vi "map_trap_switch_Stiffback.vi"() -> ()   [LabVIEW 2011]
panel:
  in  "KILL":bool
  in  "PAUSE":bool
  in  "RESUME":bool
  in  "QUIT":bool
  in  "up done":bool
  in  "z up":bool
  in  "Done":bool
  in  "z piastra":bool
  in  "y piastra":bool
  in  "x piastra":bool
  in  "goto y pos":bool
  in  "goto x pos":bool
  in  "Panello o piastre?":bool
  in  "End":bool
  in  "zero z - end":bool
  in  "zero x - end":bool
  in  "zero y - end":bool
  in  "goto z pos":bool
  in  "positioning done":bool
  out "output":string
  out "command":string
  in  "zero done":bool
  in  "zero z":bool
  in  "zero x":bool
  in  "zero y":bool
  # "Comandi di emergenza"
  # "Mappatura a trapezio \nper il pannello e le piastre\nSU STIFFBACK"
  # "In alto: TRUE ---> Panello"
  # "In basso: FALSE ---> Piastre"
  # "Posiziono in zero"
  # "Vado sulla piastra \ne azzero"
  # "Alzo il comparatore"
  # "Vado in posizione"
  # "Ritorno a zero"
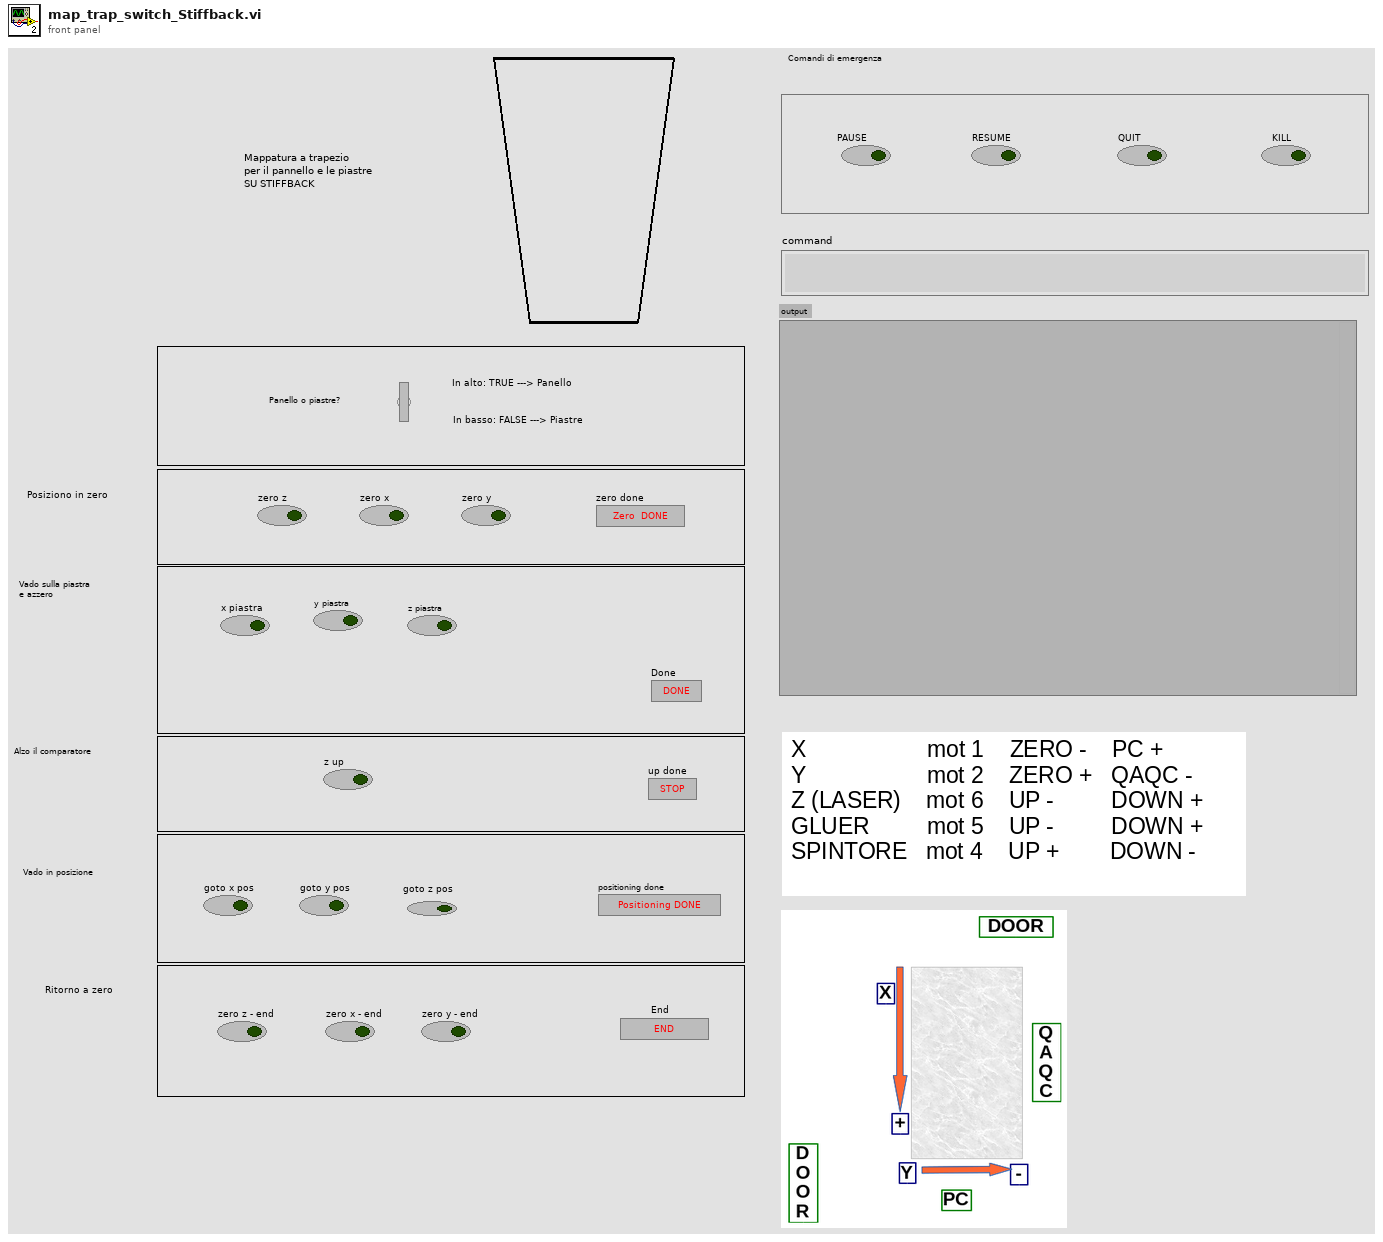
[diagram p1: front panel]
types:
  T1 = enum8{"Enabled", "Disabled", "Disabled and Grayed Out"}
  T2 = enum16{"open", "replace", "create", "open or create", "replace or create", "replace or create with confirmation"}
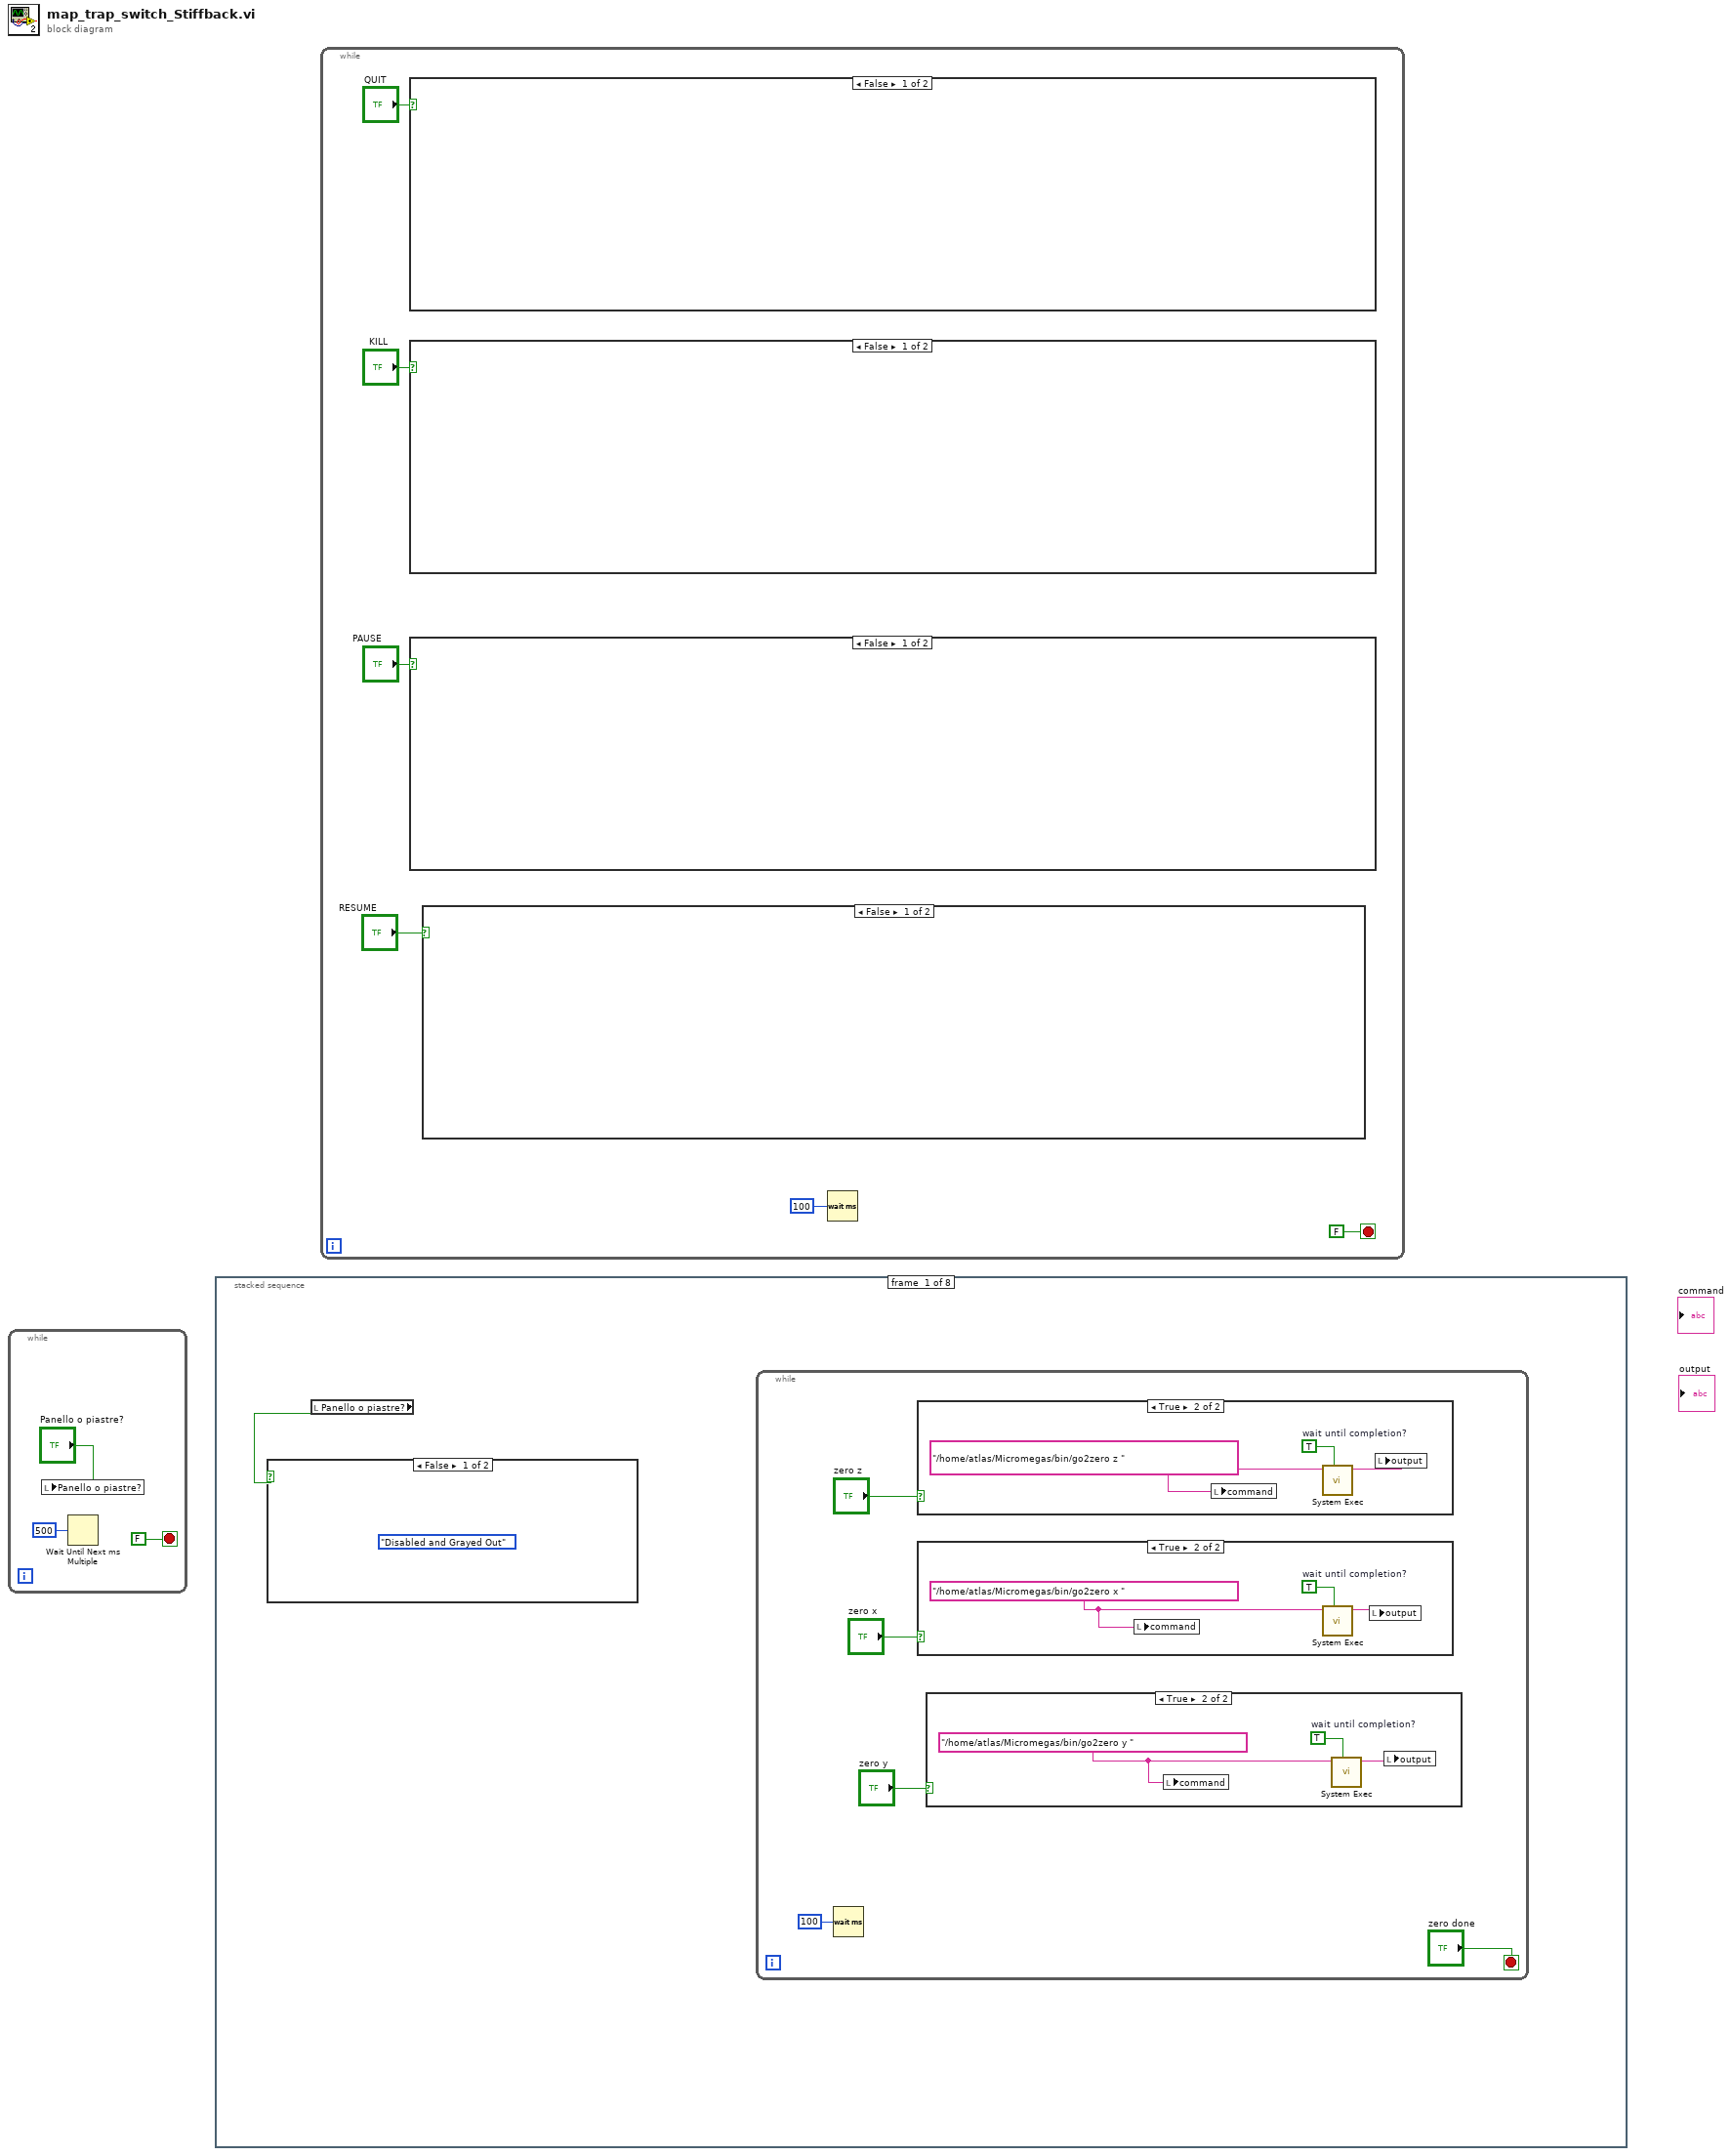
[diagram p0: block diagram]
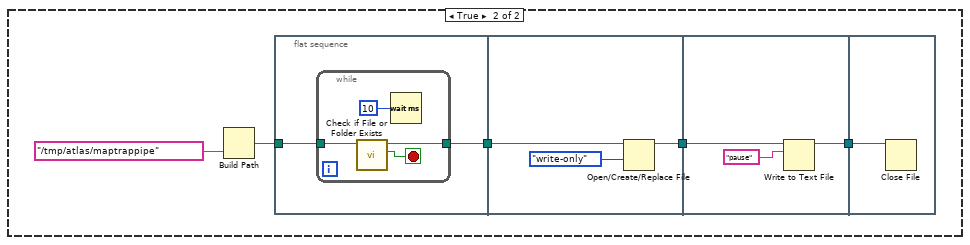
[diagram p2: hidden frame]
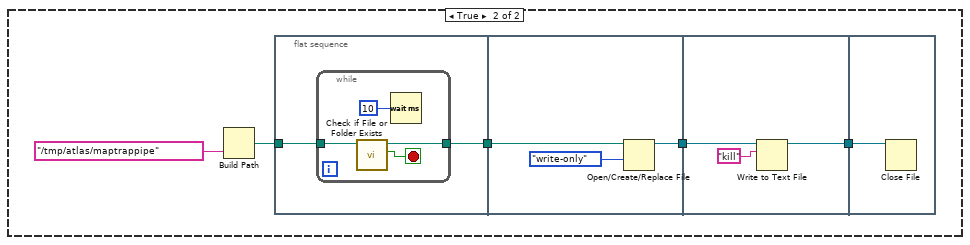
[diagram p3: hidden frame]
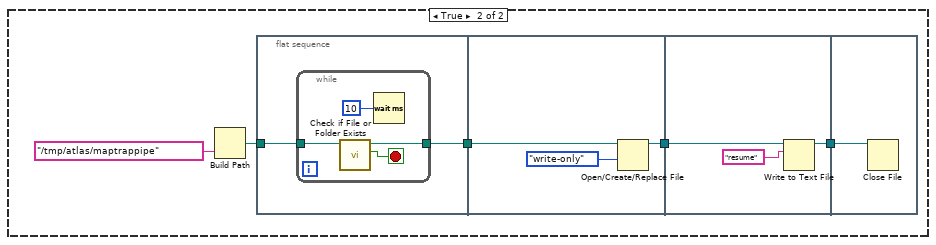
[diagram p4: hidden frame]
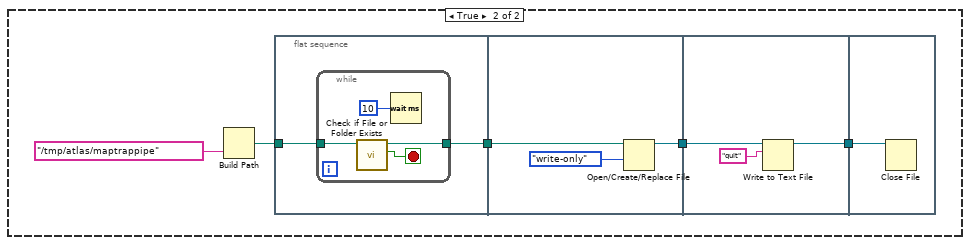
[diagram p5: hidden frame]
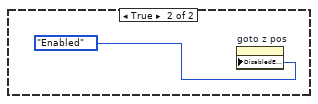
[diagram p6: hidden frame]
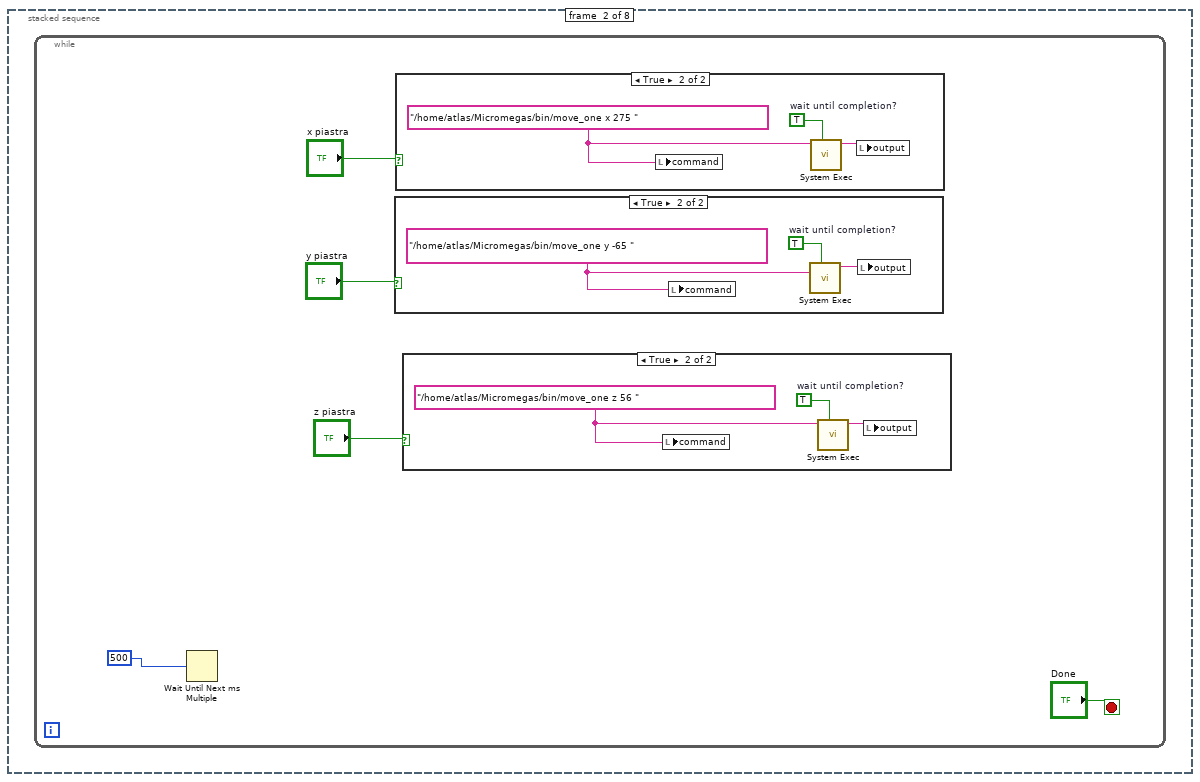
[diagram p10: hidden frame]
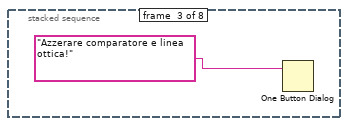
[diagram p14: hidden frame]
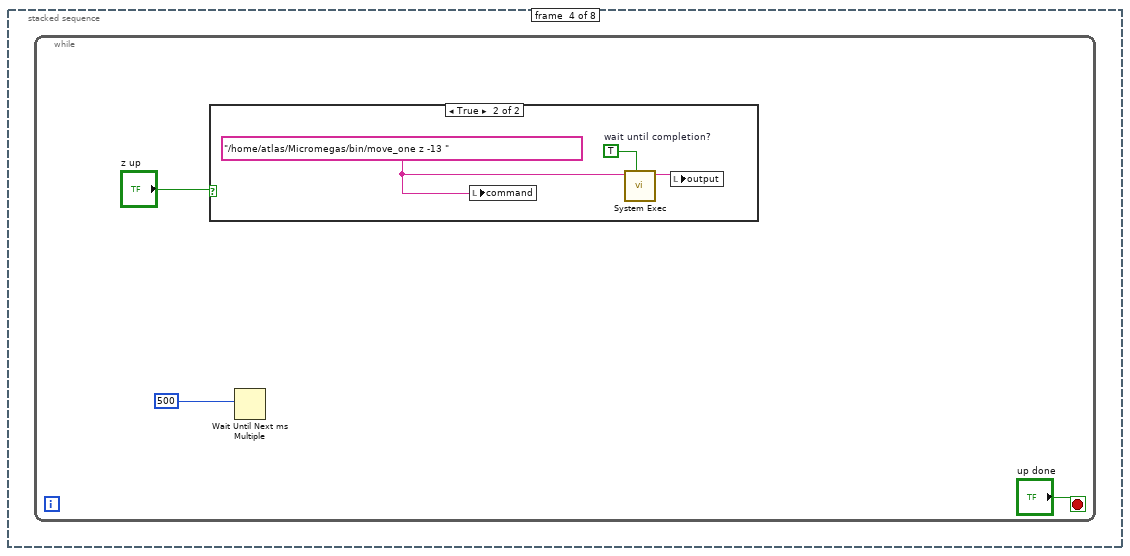
[diagram p15: hidden frame]
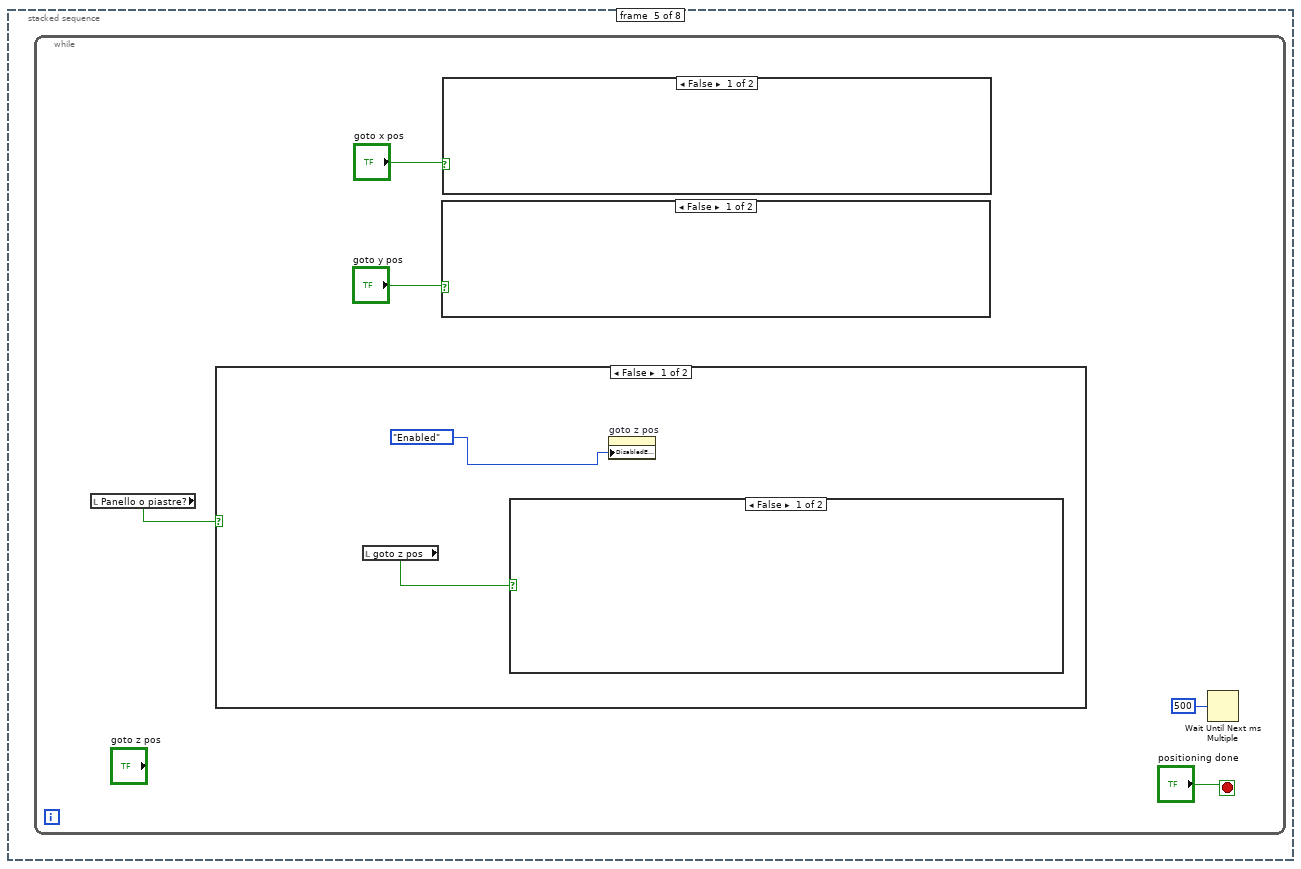
[diagram p17: hidden frame]
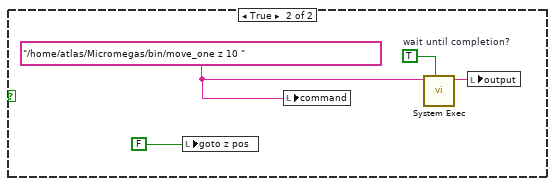
[diagram p18: hidden frame]
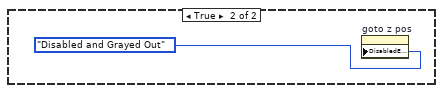
[diagram p19: hidden frame]
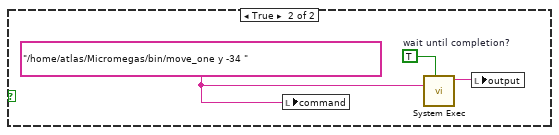
[diagram p20: hidden frame]
diagram:
  n1 = while {
    stop <- FALSE stop-if-true
    n2 = local write "Panello o piastre?"("Panello o piastre?") -> ()
    n3 = Wait Until Next ms Multiple(millisecond multiple=u32 500) -> ()  [unwired: 1 out]
  }
  n4 = stacked-sequence {
    frame #0 {
      n5 = local read "Panello o piastre?"() -> (w4:bool)
      n6 = case shown="False" w4 {
        frame False {
          (unwired) T1."Disabled and Grayed Out" ("Disabled")
        }
        frame True {
          n7 = property on="goto z pos" class="Bool (strict)"("DisabledEnum"=T1."Enabled" ("Disabled")) -> ()  [unwired: 2 in, 2 out]
        }
      }
      n8 = while {
        stop <- "zero done" stop-if-true
        n9 = Wait (ms)(milliseconds to wait=u32 100) -> ()  [unwired: 1 out]
        n10 = case shown="True" "zero z" {
          frame False {
          }
          frame True {
            w18 = "/home/atlas/Micromegas/bin/go2zero z " ("string")
            w19 = TRUE  # wait until completion?
            n11 = local write "command"(w18) -> ()
            n12 = call <vilib>:"System Exec.vi"("wait until completion? (T)"=w19, "command line"=w18) -> ("standard output"=w17:string)  [unwired: 6 in, 3 out]
            n13 = local write "output"(w17) -> ()
          }
        }
        n14 = case shown="True" "zero x" {
          frame False {
          }
          frame True {
            w15 = "/home/atlas/Micromegas/bin/go2zero x " ("string")
            w16 = TRUE  # wait until completion?
            n15 = local write "command"(w15) -> ()
            n16 = call <vilib>:"System Exec.vi"("wait until completion? (T)"=w16, "command line"=w15) -> ("standard output"=w14:string)  [unwired: 6 in, 3 out]
            n17 = local write "output"(w14) -> ()
          }
        }
        n18 = case shown="True" "zero y" {
          frame False {
          }
          frame True {
            w12 = "/home/atlas/Micromegas/bin/go2zero y " ("string")
            w13 = TRUE  # wait until completion?
            n19 = local write "command"(w12) -> ()
            n20 = call <vilib>:"System Exec.vi"("wait until completion? (T)"=w13, "command line"=w12) -> ("standard output"=w11:string)  [unwired: 6 in, 3 out]
            n21 = local write "output"(w11) -> ()
          }
        }
      }
    }
    frame #1 {
      n22 = while {
        stop <- "Done" stop-if-true
        n23 = Wait Until Next ms Multiple(millisecond multiple=u32 500 ("millisecond timer value")) -> ()  [unwired: 1 out]
        n24 = case shown="True" "y piastra" {
          frame False {
          }
          frame True {
            w28 = "/home/atlas/Micromegas/bin/move_one y -65 " ("string")
            w30 = TRUE  # wait until completion?
            n25 = local write "command"(w28) -> ()
            n26 = call <vilib>:"System Exec.vi"("wait until completion? (T)"=w30, "command line"=w28) -> ("standard output"=w29:string)  [unwired: 6 in, 3 out]
            n27 = local write "output"(w29) -> ()
          }
        }
        n28 = case shown="True" "x piastra" {
          frame False {
          }
          frame True {
            w31 = "/home/atlas/Micromegas/bin/move_one x 275 " ("string")
            w33 = TRUE  # wait until completion?
            n29 = local write "command"(w31) -> ()
            n30 = call <vilib>:"System Exec.vi"("wait until completion? (T)"=w33, "command line"=w31) -> ("standard output"=w32:string)  [unwired: 6 in, 3 out]
            n31 = local write "output"(w32) -> ()
          }
        }
        n32 = case shown="True" "z piastra" {
          frame False {
          }
          frame True {
            w25 = "/home/atlas/Micromegas/bin/move_one z 56 " ("string")
            w27 = TRUE  # wait until completion?
            n33 = local write "command"(w25) -> ()
            n34 = call <vilib>:"System Exec.vi"("wait until completion? (T)"=w27, "command line"=w25) -> ("standard output"=w26:string)  [unwired: 6 in, 3 out]
            n35 = local write "output"(w26) -> ()
          }
        }
      }
    }
    frame #2 {
      n36 = One Button Dialog(message="Azzerare comparatore e linea ottica!") -> ()  [unwired: 1 in, 1 out]
    }
    frame #3 {
      n37 = while {
        stop <- "up done" stop-if-true
        n38 = case shown="True" "z up" {
          frame False {
          }
          frame True {
            w38 = "/home/atlas/Micromegas/bin/move_one z -13 " ("string")
            w40 = TRUE  # wait until completion?
            n39 = local write "command"(w38) -> ()
            n40 = call <vilib>:"System Exec.vi"("wait until completion? (T)"=w40, "command line"=w38) -> ("standard output"=w39:string)  [unwired: 6 in, 3 out]
            n41 = local write "output"(w39) -> ()
          }
        }
        n42 = Wait Until Next ms Multiple(millisecond multiple=u32 500 ("millisecond timer value")) -> ()  [unwired: 1 out]
      }
    }
    frame #4 {
      n43 = while {
        stop <- "positioning done" stop-if-true
        n44 = local read "Panello o piastre?"() -> (w41:bool)
        n45 = case shown="False" w41 {
          frame False {
            n46 = local read "goto z pos"() -> (w47:bool)
            n47 = case shown="False" w47 {
              frame False {
              }
              frame True {
                w49 = "/home/atlas/Micromegas/bin/move_one z 10 " ("string")
                w51 = TRUE  # wait until completion?
                n48 = local write "goto z pos"(FALSE ("goto z pos")) -> ()
                n49 = local write "command"(w49) -> ()
                n50 = call <vilib>:"System Exec.vi"("wait until completion? (T)"=w51, "command line"=w49) -> ("standard output"=w50:string)  [unwired: 6 in, 3 out]
                n51 = local write "output"(w50) -> ()
              }
            }
            n52 = property on="goto z pos" class="Bool (strict)"("DisabledEnum"=T1."Enabled" ("Disabled")) -> ()  [unwired: 2 in, 2 out]
          }
          frame True {
            n53 = property on="goto z pos" class="Bool (strict)"("DisabledEnum"=T1."Disabled and Grayed Out" ("Disabled")) -> ()  [unwired: 2 in, 2 out]
          }
        }
        n54 = case shown="False" "goto y pos" {
          frame False {
          }
          frame True {
            w53 = "/home/atlas/Micromegas/bin/move_one y -34 " ("string")
            w55 = TRUE  # wait until completion?
            n55 = local write "command"(w53) -> ()
            n56 = call <vilib>:"System Exec.vi"("wait until completion? (T)"=w55, "command line"=w53) -> ("standard output"=w54:string)  [unwired: 6 in, 3 out]
            n57 = local write "output"(w54) -> ()
          }
        }
        n58 = case shown="False" "goto x pos" {
          frame False {
          }
          frame True {
            w56 = "/home/atlas/Micromegas/bin/move_one x 34 " ("string")
            w58 = TRUE  # wait until completion?
            n59 = local write "command"(w56) -> ()
            n60 = call <vilib>:"System Exec.vi"("wait until completion? (T)"=w58, "command line"=w56) -> ("standard output"=w57:string)  [unwired: 6 in, 3 out]
            n61 = local write "output"(w57) -> ()
          }
        }
        n62 = Wait Until Next ms Multiple(millisecond multiple=u32 500) -> ()  [unwired: 1 out]
      }
    }
    frame #5 {
      n63 = flat-sequence {
        frame #0 {
          n64 = Open/Create/Replace File(file path (use dialog)=path "/tmp/map_trap.tmp", operation (0:open)=T2."open or create") -> ()  [unwired: 4 in, 3 out]
          n65 = call <vilib>:"System Exec.vi"("wait until completion? (T)"=FALSE, "command line"="gnome-terminal -e \"tail -f /tmp/map_trap.tmp\"") -> ()  [unwired: 6 in, 4 out]
        }
        frame #1 {
          w69 = TRUE  # wait until completion?
          n66 = Concatenate Strings("/home/atlas/Micromegas/bin/map_trap  " ("string"), "" ("string"), "-w 2160 1120 -x 80 20 -y 80 20 -t 3 10" ("string"), "  | tee /tmp/map_trap.tmp" ("string")) -> (w64:string)
          n67 = local write "command"(w64) -> ()
          n68 = call <vilib>:"System Exec.vi"("wait until completion? (T)"=w69, "command line"=w64) -> ("standard output"=w63:string)  [unwired: 6 in, 3 out]
          n69 = local write "output"(w63) -> ()
        }
      }
    }
    frame #6 {
      n70 = while {
        stop <- "End" stop-if-true
        n71 = Wait (ms)(milliseconds to wait=u32 100) -> ()  [unwired: 1 out]
        n72 = case shown="True" "zero z - end" {
          frame False {
          }
          frame True {
            w82 = "/home/atlas/Micromegas/bin/go2zero z " ("string")
            w83 = TRUE  # wait until completion?
            n73 = local write "command"(w82) -> ()
            n74 = call <vilib>:"System Exec.vi"("wait until completion? (T)"=w83, "command line"=w82) -> ("standard output"=w81:string)  [unwired: 6 in, 3 out]
            n75 = local write "output"(w81) -> ()
          }
        }
        n76 = case shown="True" "zero x - end" {
          frame False {
          }
          frame True {
            w79 = "/home/atlas/Micromegas/bin/go2zero x " ("string")
            w80 = TRUE  # wait until completion?
            n77 = local write "command"(w79) -> ()
            n78 = call <vilib>:"System Exec.vi"("wait until completion? (T)"=w80, "command line"=w79) -> ("standard output"=w78:string)  [unwired: 6 in, 3 out]
            n79 = local write "output"(w78) -> ()
          }
        }
        n80 = case shown="True" "zero y - end" {
          frame False {
          }
          frame True {
            w76 = "/home/atlas/Micromegas/bin/go2zero y " ("string")
            w77 = TRUE  # wait until completion?
            n81 = local write "command"(w76) -> ()
            n82 = call <vilib>:"System Exec.vi"("wait until completion? (T)"=w77, "command line"=w76) -> ("standard output"=w75:string)  [unwired: 6 in, 3 out]
            n83 = local write "output"(w75) -> ()
          }
        }
      }
    }
    frame #7 {
      n84 = One Button Dialog(message="Per comodita`, rinominare il file (non verra` comunque sovrascritto)") -> ()  [unwired: 1 in, 1 out]
    }
  }
  n85 = while {
    stop <- FALSE stop-if-true
    n86 = case shown="False" "QUIT" {
      frame False {
      }
      frame True {
        n87 = Build Path(name or relative path="/tmp/atlas/maptrappipe" ("string")) -> (appended path=w145:path)  [unwired: 1 in]
        n88 = flat-sequence {
          tunnel: [w151] -> w149
          tunnel: w145 -> [w150]
          tunnel: w149 -> [w158]
          tunnel: [w156] -> w148
          tunnel: w148 -> [w161]
          tunnel: [w160] -> w147
          tunnel: w147 -> [w162]
          frame #0 {
            n89 = while {
              tunnel: [w153] -> w151
              tunnel: w150 -> [w152]
              stop <- w154 stop-if-true
              n90 = call <vilib>:"Check if File or Folder Exists.vi"("path"=w152) -> ("file or folder exists?"=w154:bool, "dup path"=w153:path)  [unwired: 8 in, 1 out]
              n91 = Wait (ms)(milliseconds to wait=u32 10) -> ()  [unwired: 1 out]
            }
          }
          frame #1 {
            n92 = Open/Create/Replace File(file path (use dialog)=w158, access (0:read/write)=enum16{"read/write", "read-only", "write-only"}."write-only") -> (refnum out=w156:refnum<file>)  [unwired: 4 in, 2 out]
          }
          frame #2 {
            n93 = Write to Text File(file (use dialog)=w161, text="quit") -> (refnum out=w160:refnum<file>)  [unwired: 2 in, 2 out]
          }
          frame #3 {
            n94 = Close File(refnum=w162) -> ()  [unwired: 1 in, 2 out]
          }
        }
      }
    }
    n95 = case shown="False" "KILL" {
      frame False {
      }
      frame True {
        n96 = Build Path(name or relative path="/tmp/atlas/maptrappipe" ("string")) -> (appended path=w109:path)  [unwired: 1 in]
        n97 = flat-sequence {
          tunnel: [w115] -> w113
          tunnel: w109 -> [w114]
          tunnel: w113 -> [w122]
          tunnel: [w120] -> w112
          tunnel: w112 -> [w125]
          tunnel: [w124] -> w111
          tunnel: w111 -> [w126]
          frame #0 {
            n98 = while {
              tunnel: [w117] -> w115
              tunnel: w114 -> [w116]
              stop <- w118 stop-if-true
              n99 = call <vilib>:"Check if File or Folder Exists.vi"("path"=w116) -> ("file or folder exists?"=w118:bool, "dup path"=w117:path)  [unwired: 8 in, 1 out]
              n100 = Wait (ms)(milliseconds to wait=u32 10) -> ()  [unwired: 1 out]
            }
          }
          frame #1 {
            n101 = Open/Create/Replace File(file path (use dialog)=w122, access (0:read/write)=enum16{"read/write", "read-only", "write-only"}."write-only") -> (refnum out=w120:refnum<file>)  [unwired: 4 in, 2 out]
          }
          frame #2 {
            n102 = Write to Text File(file (use dialog)=w125, text="kill") -> (refnum out=w124:refnum<file>)  [unwired: 2 in, 2 out]
          }
          frame #3 {
            n103 = Close File(refnum=w126) -> ()  [unwired: 1 in, 2 out]
          }
        }
      }
    }
    n104 = case shown="False" "PAUSE" {
      frame False {
      }
      frame True {
        n105 = Build Path(name or relative path="/tmp/atlas/maptrappipe" ("string")) -> (appended path=w91:path)  [unwired: 1 in]
        n106 = flat-sequence {
          tunnel: [w97] -> w95
          tunnel: w91 -> [w96]
          tunnel: w95 -> [w104]
          tunnel: [w102] -> w94
          tunnel: w94 -> [w107]
          tunnel: [w106] -> w93
          tunnel: w93 -> [w108]
          frame #0 {
            n107 = while {
              tunnel: [w99] -> w97
              tunnel: w96 -> [w98]
              stop <- w100 stop-if-true
              n108 = call <vilib>:"Check if File or Folder Exists.vi"("path"=w98) -> ("file or folder exists?"=w100:bool, "dup path"=w99:path)  [unwired: 8 in, 1 out]
              n109 = Wait (ms)(milliseconds to wait=u32 10) -> ()  [unwired: 1 out]
            }
          }
          frame #1 {
            n110 = Open/Create/Replace File(file path (use dialog)=w104, access (0:read/write)=enum16{"read/write", "read-only", "write-only"}."write-only") -> (refnum out=w102:refnum<file>)  [unwired: 4 in, 2 out]
          }
          frame #2 {
            n111 = Write to Text File(file (use dialog)=w107, text="pause") -> (refnum out=w106:refnum<file>)  [unwired: 2 in, 2 out]
          }
          frame #3 {
            n112 = Close File(refnum=w108) -> ()  [unwired: 1 in, 2 out]
          }
        }
      }
    }
    n113 = case shown="False" "RESUME" {
      frame False {
      }
      frame True {
        n114 = Build Path(name or relative path="/tmp/atlas/maptrappipe" ("string")) -> (appended path=w127:path)  [unwired: 1 in]
        n115 = flat-sequence {
          tunnel: [w133] -> w131
          tunnel: w127 -> [w132]
          tunnel: w131 -> [w140]
          tunnel: [w138] -> w130
          tunnel: w130 -> [w143]
          tunnel: [w142] -> w129
          tunnel: w129 -> [w144]
          frame #0 {
            n116 = while {
              tunnel: [w135] -> w133
              tunnel: w132 -> [w134]
              stop <- w136 stop-if-true
              n117 = call <vilib>:"Check if File or Folder Exists.vi"("path"=w134) -> ("file or folder exists?"=w136:bool, "dup path"=w135:path)  [unwired: 8 in, 1 out]
              n118 = Wait (ms)(milliseconds to wait=u32 10) -> ()  [unwired: 1 out]
            }
          }
          frame #1 {
            n119 = Open/Create/Replace File(file path (use dialog)=w140, access (0:read/write)=enum16{"read/write", "read-only", "write-only"}."write-only") -> (refnum out=w138:refnum<file>)  [unwired: 4 in, 2 out]
          }
          frame #2 {
            n120 = Write to Text File(file (use dialog)=w143, text="resume") -> (refnum out=w142:refnum<file>)  [unwired: 2 in, 2 out]
          }
          frame #3 {
            n121 = Close File(refnum=w144) -> ()  [unwired: 1 in, 2 out]
          }
        }
      }
    }
    n122 = Wait (ms)(milliseconds to wait=100) -> ()  [unwired: 1 out]
  }
